vi "Cursor Demo 1.vi"() -> ()   [LabVIEW 2016]
panel:
  in  "Boolean":bool
  in  "Slide":dbl(slide) scale=0.0..20.0
  out "Waveform Graph":dbl[](graph)
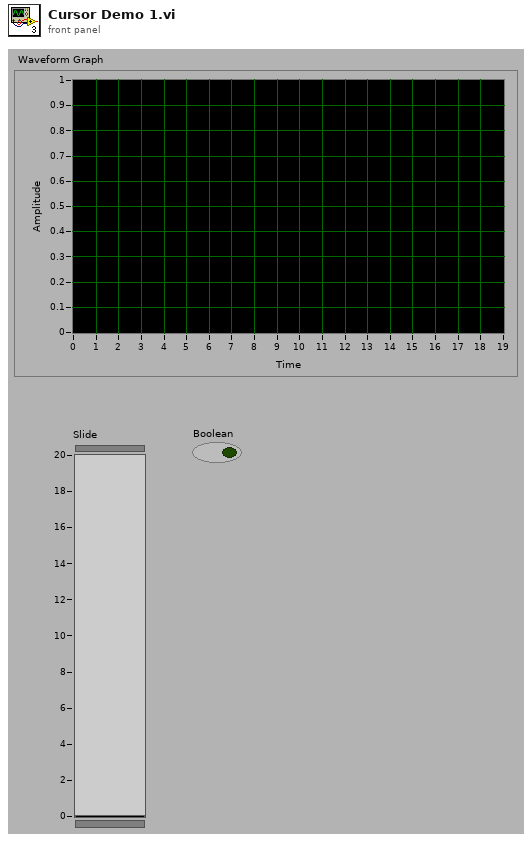
[diagram p1: front panel]
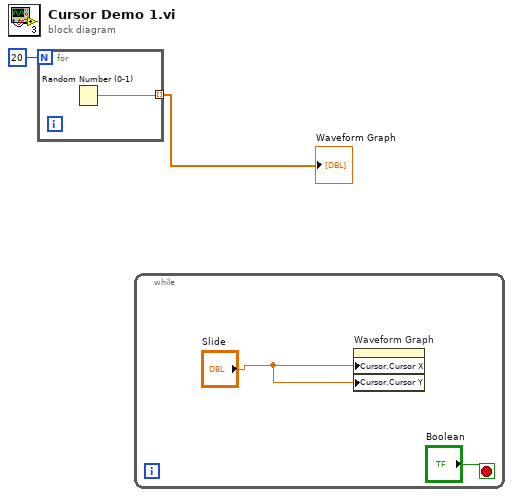
[diagram p0: block diagram]
diagram:
  n1 = for {
    N: 20 -> [_]
    tunnel: [w3] -> w1 mode=indexing
    n2 = Random Number (0-1)() -> (number: 0 to 1=w3:dbl)
  }
  "Waveform Graph" <- w1
  n3 = while {
    stop <- "Boolean" stop-if-true
    n4 = property on="Waveform Graph" class="WFGraph (strict)"("Cursor.Cursor X"="Slide", "Cursor.Cursor Y"="Slide") -> ()  [unwired: 2 in, 2 out]
  }
